vi "rsscope_core_global.vi"() -> ()   [LabVIEW 2018] (continued)
 matches Phase_seg2 specified in the CAN standard.\n\nNote: The maximum sum of Time segment 1 and Time segment 2 is 24.\n\nRemote-control command(s):\nBUS<m>:CAN:T1Segment\nBUS<m>:CAN:T2Segment\n\nAvailable Repeated Capabilities:\nSerialBus: SB1, SB2, SB3, SB4\r\nCANTimeSeg: TS1, TS2\r\n\nRemote-control command(s):\nBUS<m>:CAN:T<CANTimeSeg>Segment"}, {"Level"=4, "Class Only"=FALSE, "Identifier"="RSSCOPE_ATTR_PROTOCOL_CAN_FD_SAMPLE_POINT_ABS", "Descriptive Name"="Protocol CAN FD Sample Point Abs", "Data Type"=0, "Command"="BUS{SerialBus}:CAN:FDAT:T{CANTimeSeg}S", "Access"=2, "Range Table"="RsScope_rngProtocolCANSamplePointAbs", "Read Callback"="", "Write Callback"="", "Supported Models"="", "Instrument Options"="K0|K3", "Flags"=0, "Help"="Set the number of time quanta before the sample point (T1Segment) and after the sample point (T2Segment). T1Segment comprises the segments Synch_seg, Prop_seg, and Phase_seg1 which are specified in the CAN standard. T2Segment matches Phase_seg2 specified in the CAN standard.\n\nNote: The maximum sum of Time segment 1 and Time segment 2 is 24.\n\nRemote-control command(s):\nBUS<m>:CAN:FDATa:T1Segment\nBUS<m>:CAN:FDATa:T2Segment\n\nAvailable Repeated Capabilities:\nSerialBus: SB1, SB2, SB3, SB4\r\nCANTimeSeg: TS1, TS2\r\n\nRemote-control command(s):\nBUS<m>:CAN:FDATa:T<CANTimeSeg>Segment"}, {"Level"=2, "Class Only"=TRUE, "Identifier"="", "Descriptive Name"="FlexRay", "Data Type"=0, "Command"="", "Access"=0, "Range Table"="", "Read Callback"="", "Write Callback"="", "Supported Models"="", "Instrument Options"="", "Flags"=0, "Help"="FlexRay is designed for use in safety-related distributed applications in the automotive industry. It is applied in real-time applications when higher data rates and reliable communication are required. In particular, FlexRay supports x-by-wire applications, e.g. steer-by-wire or brake-by-wire.\n\nAttributes in this class require option R&S RTO-K3."}, {"Level"=3, "Class Only"=FALSE, "Identifier"="RSSCOPE_ATTR_PROTOCOL_FLEXRAY_SOURCE_TYPE", "Descriptive Name"="Protocol FlexRay Source Type", "Data Type"=0, "Command"="BUS{SerialBus}:FLXR:SRCT", "Access"=2, "Range Table"="rsscope_rngFlexRaySrcType", "Read Callback"="", "Write Callback"="", "Supported Models"="", "Instrument Options"="K4", "Flags"=0, "Help"="Selects the FlexRay source type.\n\nAvailable Repeated Capabilities:\nSerialBus: SB1, SB2, SB3, SB4\r\n\nRemote-control command(s):\nBUS<m>:FLXRay:SRCType"}, {"Level"=3, "Class Only"=FALSE, "Identifier"="RSSCOPE_ATTR_PROTOCOL_FLEXRAY_SINGLE_POLARITY", "Descriptive Name"="Protocol FlexRay Single Polarity", "Data Type"=0, "Command"="BUS{SerialBus}:FLXR:POL", "Access"=2, "Range Table"="rsscope_rngFlexRayPolarity", "Read Callback"="", "Write Callback"="", "Supported Models"="", "Instrument Options"="K4", "Flags"=0, "Help"="Selects the wire on which the bus signal is  measured in case of SINGle source type. The setting affects the digitization of the signal.\n\nAvailable Repeated Capabilities:\nSerialBus: SB1, SB2, SB3, SB4\r\n\nRemote-control command(s):\nBUS<m>:FLXRay:POLarity"}, {"Level"=3, "Class Only"=FALSE, "Identifier"="RSSCOPE_ATTR_PROTOCOL_FLEXRAY_SINGLE_PRESET_TRESHOLD", "Descriptive Name"="Protocol FlexRay Single Preset Treshold", "Data Type"=0, "Command"="BUS{SerialBus}:FLXR:PRS", "Access"=2, "Range Table"="rsscope_rngFlexRaySinglePreset", "Read Callback"="", "Write Callback"="", "Supported Models"="", "Instrument Options"="K4", "Flags"=0, "Help"="This control selecs a default threshold voltage.\n\nAvailable Repeated Capabilities:\nSerialBus: SB1, SB2, SB3, SB4\r\n\nRemote-control command(s):\nBUS<m>:FLXRay:PRSingle"}, {"Level"=3, "Class Only"=FALSE, "Identifier"="RSSCOPE_ATTR_PROTOCOL_FLEXRAY_DIFF_PRESET_TRESHOLD", "Descriptive Name"="Protocol FlexRay Differential Preset Treshold", "Data Type"=0, "Command"="BUS{SerialBus}:FLXR:PRD", "Access"=2, "Range Table"="rsscope_rngFlexRayDifferentialPreset", "Read Callback"="", "Write Callback"="", "Supported Models"="", "Instrument Options"="K4", "Flags"=0, "Help"="Selecs a default threshold voltage.\n\nAvailable Repeated Capabilities:\nSerialBus: SB1, SB2, SB3, SB4\r\n\nRemote-control command(s):\nBUS<m>:FLXRay:PRDiff"}, {"Level"=3, "Class Only"=FALSE, "Identifier"="RSSCOPE_ATTR_PROTOCOL_FLEXRAY_THRESHOLD_HIGH", "Descriptive Name"="Protocol FlexRay Threshold High", "Data Type"=1, "Command"="BUS{SerialBus}:FLXR:THR1", "Access"=2, "Range Table"="", "Read Callback"="", "Write Callback"="", "Supported Models"="", "Instrument Options"="K4", "Flags"=0, "Help"="Sets the thresholds for the bus signal if the source type is Single or Differential.\n\nAvailable Repeated Capabilities:\nSerialBus: SB1, SB2, SB3, SB4\r\n\nRemote-control command(s):\nBUS<m>:FLXRay:THReshold<n>"}, {"Level"=3, "Class Only"=FALSE, "Identifier"="RSSCOPE_ATTR_PROTOCOL_FLEXRAY_THRESHOLD_LOW", "Descriptive Name"="Protocol FlexRay Threshold Low", "Data Type"=1, "Command"="BUS{SerialBus}:FLXR:THR2", "Access"=2, "Range Table"="", "Read Callback"="", "Write Callback"="", "Supported Models"="", "Instrument Options"="K4", "Flags"=0, "Help"="Sets the thresholds for the bus signal if the source type is Single or Differential.\n\nAvailable Repeated Capabilities:\nSerialBus: SB1, SB2, SB3, SB4\r\n\nRemote-control command(s):\nBUS<m>:FLXRay:THReshold<n>"}, {"Level"=3, "Class Only"=FALSE, "Identifier"="RSSCOPE_ATTR_PROTOCOL_FLEXRAY_LOGIC_PRESET_TRESHOLD", "Descriptive Name"="Protocol FlexRay Logic Preset Treshold", "Data Type"=0, "Command"="BUS{SerialBus}:FLXR:PRL", "Access"=2, "Range Table"="rsscope_rngFlexRayLogicPreset", "Read Callback"="", "Write Callback"="", "Supported Models"="", "Instrument Options"="K4", "Flags"=0, "Help"="This attribute selecs a default threshold voltage.\n\nAvailable Repeated Capabilities:\nSerialBus: SB1, SB2, SB3, SB4\r\n\nRemote-control command(s):\nBUS<m>:FLXRay:PRLogic"}, {"Level"=3, "Class Only"=FALSE, "Identifier"="RSSCOPE_ATTR_PROTOCOL_FLEXRAY_THRESHOLD_DATA", "Descriptive Name"="Protocol FlexRay Threshold Data", "Data Type"=1, "Command"="BUS{SerialBus}:FLXR:THD", "Access"=2, "Range Table"="rsscope_rngFlexRayLogicTreshold", "Read Callback"="", "Write Callback"="", "Supported Models"="", "Instrument Options"="", "Flags"=0, "Help"="Sets the threshold for the data line if the source type is LOGic.\n\nAvailable Repeated Capabilities:\nSerialBus: SB1, SB2, SB3, SB4\r\n\nRemote-control command(s):\nBUS<m>:FLXRay:THData"}, {"Level"=3, "Class Only"=FALSE, "Identifier"="RSSCOPE_ATTR_PROTOCOL_FLEXRAY_THRESHOLD_ENABLE", "Descriptive Name"="Protocol FlexRay Threshold Enable", "Data Type"=1, "Command"="BUS{SerialBus}:FLXR:THEN", "Access"=2, "Range Table"="rsscope_rngFlexRayLogicTreshold", "Read Callback"="", "Write Callback"="", "Supported Models"="", "Instrument Options"="", "Flags"=0, "Help"="Sets the threshold for the enable line if the source type is LOGic.\n\nAvailable Repeated Capabilities:\nSerialBus: SB1, SB2, SB3, SB4\r\n\nRemote-control command(s):\nBUS<m>:FLXRay:THENable"}, {"Level"=3, "Class Only"=FALSE, "Identifier"="RSSCOPE_ATTR_PROTOCOL_FLEXRAY_BIT_RATE", "Descriptive Name"="Protocol FlexRay Bit Rate", "Data Type"=0, "Command"="BUS{SerialBus}:FLXR:BITR", "Access"=2, "Range Table"="rsscope_rngFlexRayBitRate", "Read Callback"="", "Write Callback"="", "Supported Models"="", "Instrument Options"="", "Flags"=0, "Help"="Selects the bit rate.\n\nAvailable Repeated Capabilities:\nSerialBus: SB1, SB2, SB3, SB4\r\n\nRemote-control command(s):\nBUS<m>:FLXRay:BITRate"}, {"Level"=3, "Class Only"=FALSE, "Identifier"="RSSCOPE_ATTR_PROTOCOL_FLEXRAY_CHANNEL", "Descriptive Name"="Protocol FlexRay Channel", "Data Type"=0, "Command"="BUS{SerialBus}:FLXR:CHTY", "Access"=2, "Range Table"="rsscope_rngFlexRayChannel", "Read Callback"="", "Write Callback"="", "Supported Models"="", "Instrument Options"="K4", "Flags"=0, "Help"="Selects the channel on which the signal is measured. The setting is considered in the calculation of the frame CRC.\n\nAvailable Repeated Capabilities:\nSerialBus: SB1, SB2, SB3, SB4\r\n\nRemote-control command(s):\nBUS<m>:FLXRay:CHTYpe"}, {"Level"=3, "Class Only"=FALSE, "Identifier"="RSSCOPE_ATTR_PROTOCOL_FLEXRAY_SEPARATE_HEADER_BITS", "Descriptive Name"="Protocol FlexRay Separate Header Bits", "Data Type"=3, "Command"="BUS{SerialBus}:FLXR:SEHB", "Access"=2, "Range Table"="", "Read Callback"="", "Write Callback"="", "Supported Models"="", "Instrument Options"="K4", "Flags"=0, "Help"="Affects the decoding and its display. If ON, the leading five indicator bits of the header are decoded as five single bits. Otherwise, the indicator bits are shown as one word with word length five bit.\n\nAvailable Repeated Capabilities:\nSerialBus: SB1, SB2, SB3, SB4\r\n\nRemote-control command(s):\nBUS<m>:FLXRay:SEHB"}, {"Level"=3, "Class Only"=FALSE, "Identifier"="RSSCOPE_ATTR_PROTOCOL_FLEXRAY_SELECTED_FRAME", "Descriptive Name"="Protocol FlexRay Selected Frame", "Data Type"=0, "Command"="", "Access"=2, "Range Table"="", "Read Callback"="", "Write Callback"="", "Supported Models"="", "Instrument Options"="", "Flags"=0, "Help"="Sets selector repeated capability Frame.\n\nAvailable Repeated Capabilities:\nNone\n\nRemote-control command(s):\ncmd"}, {"Level"=3, "Class Only"=FALSE, "Identifier"="RSSCOPE_ATTR_PROTOCOL_FLEXRAY_FRAME_COUNT", "Descriptive Name"="Protocol FlexRay Frame Count", "Data Type"=0, "Command"="BUS{SerialBus}:FLXR:FCO?", "Access"=0, "Range Table"="", "Read Callback"="", "Write Callback"="", "Supported Models"="", "Instrument Options"="K4", "Flags"=0, "Help"="Queries the number of decoded frames.\n\nAvailable Repeated Capabilities:\nSerialBus: SB1, SB2, SB3, SB4\r\n\nRemote-control command(s):\nBUS<m>:FLXRay:FCOunt?"}, {"Level"=3, "Class Only"=FALSE, "Identifier"="RSSCOPE_ATTR_PROTOCOL_FLEXRAY_FRAME_STATUS", "Descriptive Name"="Protocol FlexRay Frame Status", "Data Type"=0, "Command"="BUS{SerialBus}:FLXR:FRAM<Frame>:STAT?", "Access"=0, "Range Table"="rsscope_rngFlexRayFrameStatus", "Read Callback"="rsscope_FormatFlexRayFrameRepCapInt32_ReadCallback.vi", "Write Callback"="", "Supported Models"="", "Instrument Options"="K4", "Flags"=0, "Help"="Returns the overall state of the frame.\n\nAvailable Repeated Capabilities:\nSerialBus: SB1, SB2, SB3, SB4\r\n\nRemote-control command(s):\nBUS<m>:FLXRay:FRAMe<n>:STATus?"}, {"Level"=3, "Class Only"=FALSE, "Identifier"="RSSCOPE_ATTR_PROTOCOL_FLEXRAY_FRAME_START", "Descriptive Name"="Protocol FlexRay Frame Start", "Data Type"=1, "Command"="BUS{SerialBus}:FLXR:FRAM<Frame>:STAR?", "Access"=0, "Range Table"="", "Read Callback"="rsscope_FormatFlexRayFrameRepCapReal64_ReadCallback.vi", "Write Callback"="", "Supported Models"="", "Instrument Options"="K4", "Flags"=0, "Help"="Return the start time of the selected frame.\n\nAvailable Repeated Capabilities:\nSerialBus: SB1, SB2, SB3, SB4\r\n\nRemote-control command(s):\nBUS<m>:FLXRay:FRAMe<n>:STARt?"}, {"Level"=3, "Class Only"=FALSE, "Identifier"="RSSCOPE_ATTR_PROTOCOL_FLEXRAY_FRAME_STOP", "Descriptive Name"="Protocol FlexRay Frame Stop", "Data Type"=1, "Command"="BUS{SerialBus}:FLXR:FRAM<Frame>:STOP?", "Access"=0, "Range Table"="", "Read Callback"="rsscope_FormatFlexRayFrameRepCapReal64_ReadCallback.vi", "Write Callback"="", "Supported Models"="", "Instrument Options"="K4", "Flags"=0, "Help"="Return the stop time of the selected frame.\n\nAvailable Repeated Capabilities:\nSerialBus: SB1, SB2, SB3, SB4\r\n\nRemote-control command(s):\nBUS<m>:FLXRay:FRAMe<n>:STOP?"}, {"Level"=3, "Class Only"=FALSE, "Identifier"="RSSCOPE_ATTR_PROTOCOL_FLEXRAY_FRAME_TYPE", "Descriptive Name"="Protocol FlexRay Frame Type", "Data Type"=0, "Command"="BUS{SerialBus}:FLXR:FRAM<Frame>:TYPE?", "Access"=0, "Range Table"="rsscope_rngFlexRayFrameType", "Read Callback"="rsscope_FormatFlexRayFrameRepCapInt32_ReadCallback.vi", "Write Callback"="", "Supported Models"="", "Instrument Options"="K4", "Flags"=0, "Help"="Returns the frame type of the selected frame.\n\nAvailable Repeated Capabilities:\nSerialBus: SB1, SB2, SB3, SB4\r\n\nRemote-control command(s):\nBUS<m>:FLXRay:FRAMe<n>:TYPE?"}, {"Level"=3, "Class Only"=FALSE, "Identifier"="RSSCOPE_ATTR_PROTOCOL_FLEXRAY_FRAME_FLAGS", "Descriptive Name"="Protocol FlexRay Frame Flags", "Data Type"=0, "Command"="BUS{SerialBus}:FLXR:FRAM<Frame>:FLAG?", "Access"=0, "Range Table"="", "Read Callback"="rsscope_FormatFlexRayFrameRepCapInt32_ReadCallback.vi", "Write Callback"="", "Supported Models"="", "Instrument Options"="K4", "Flags"=0, "Help"="Returns the value of the indicator bits at the beginning of the header segment. The five bits are read as one word.\n\nAvailable Repeated Capabilities:\nSerialBus: SB1, SB2, SB3, SB4\r\n\nRemote-control command(s):\nBUS<m>:FLXRay:FRAMe<n>:FLAGs?"}, {"Level"=3, "Class Only"=FALSE, "Identifier"="RSSCOPE_ATTR_PROTOCOL_FLEXRAY_FRAME_PAYLOAD_LENGTH", "Descriptive Name"="Protocol FlexRay Frame Payload Length", "Data Type"=0, "Command"="BUS{SerialBus}:FLXR:FRAM<Frame>:PAYL?", "Access"=0, "Range Table"="", "Read Callback"="rsscope_FormatFlexRayFrameRepCapInt32_ReadCallback.vi", "Write Callback"="", "Supported Models"="", "Instrument Options"="K4", "Flags"=0, "Help"="Returns the payload length, the number of data words in the payload segment. Information is transmitted in 2-byte words, so the number of data bytes in the payload segment is twice the payload length.\n\nAvailable Repeated Capabilities:\nSerialBus: SB1, SB2, SB3, SB4\r\n\nRemote-control command(s):\nBUS<m>:FLXRay:FRAMe<n>:PAYLength?"}, {"Level"=3, "Class Only"=FALSE, "Identifier"="RSSCOPE_ATTR_PROTOCOL_FLEXRAY_FRAME_IDENTIFIER", "Descriptive Name"="Protocol FlexRay Frame Identifier", "Data Type"=0, "Command"="BUS{SerialBus}:FLXR:FRAM<Frame>:ADID?", "Access"=0, "Range Table"="", "Read Callback"="rsscope_FormatFlexRayFrameRepCapInt32_ReadCallback.vi", "Write Callback"="", "Supported Models"="", "Instrument Options"="K4", "Flags"=0, "Help"="Returns the frame identifier, the number of the slot in which the frame is transmitted.\n\nAvailable Repeated Capabilities:\nSerialBus: SB1, SB2, SB3, SB4\r\n\nRemote-control command(s):\nBUS<m>:FLXRay:FRAMe<n>:ADID?"}, {"Level"=3, "Class Only"=FALSE, "Identifier"="RSSCOPE_ATTR_PROTOCOL_FLEXRAY_FRAME_HEADER_CRC", "Descriptive Name"="Protocol FlexRay Frame Header CRC", "Data Type"=0, "Command"="BUS{SerialBus}:FLXR:FRAM<Frame>:CSV?", "Access"=0, "Range Table"="", "Read Callback"="rsscope_FormatFlexRayFrameRepCapInt32_ReadCallback.vi", "Write Callback"="", "Supported Models"="", "Instrument Options"="K4", "Flags"=0, "Help"="Returns the cyclic redundancy check code of the frame CRC.\n\nAvailable Repeated Capabilities:\nSerialBus: SB1, SB2, SB3, SB4\r\n\nRemote-control command(s):\nBUS<m>:FLXRay:FRAMe<n>:CSValue?"}, {"Level"=3, "Class Only"=FALSE, "Identifier"="RSSCOPE_ATTR_PROTOCOL_FLEXRAY_FRAME_CRC", "Descriptive Name"="Protocol FlexRay Frame CRC", "Data Type"=0, "Command"="BUS{SerialBus}:FLXR:FRAM<Frame>:FCV?", "Access"=0, "Range Table"="", "Read Callback"="rsscope_FormatFlexRayFrameRepCapInt32_ReadCallback.vi", "Write Callback"="", "Supported Models"="", "Instrument Options"="K4", "Flags"=0, "Help"="Returns the checksum value of the header CRC.\n\nAvailable Repeated Capabilities:\nSerialBus: SB1, SB2, SB3, SB4\r\n\nRemote-control command(s):\nBUS<m>:FLXRay:FRAMe<n>:FCValue?"}, {"Level"=3, "Class Only"=FALSE, "Identifier"="RSSCOPE_ATTR_PROTOCOL_FLEXRAY_FRAME_HEADER_CRC_STATUS", "Descriptive Name"="Protocol FlexRay Frame Header CRC Status", "Data Type"=0, "Command"="BUS{SerialBus}:FLXR:FRAM<Frame>:CSST?", "Access"=0, "Range Table"="rsscope_rngFlexRayFieldStatus", "Read Callback"="rsscope_FormatFlexRayFrameRepCapInt32_ReadCallback.vi", "Write Callback"="", "Supported Models"="", "Instrument Options"="K4", "Flags"=0, "Help"="Returns the state of the cyclic redundancy check code of the frame data.\n\nAvailable Repeated Capabilities:\nSerialBus: SB1, SB2, SB3, SB4\r\n\nRemote-control command(s):\nBUS<m>:FLXRay:FRAMe<n>:CSSTate?"}, {"Level"=3, "Class Only"=FALSE, "Identifier"="RSSCOPE_ATTR_PROTOCOL_FLEXRAY_FRAME_CRC_STATUS", "Descriptive Name"="Protocol FlexRay Frame CRC Status", "Data Type"=0, "Command"="BUS{SerialBus}:FLXR:FRAM<Frame>:FCST?", "Access"=0, "Range Table"="rsscope_rngFlexRayFieldStatus", "Read Callback"="rsscope_FormatFlexRayFrameRepCapInt32_ReadCallback.vi", "Write Callback"="", "Supported Models"="", "Instrument Options"="K4", "Flags"=0, "Help"="Returns the state of the cyclic redundancy check code of the header data.\n\nAvailable Repeated Capabilities:\nSerialBus: SB1, SB2, SB3, SB4\r\n\nRemote-control command(s):\nBUS<m>:FLXRay:FRAMe<n>:FCSTate?"}, {"Level"=3, "Class Only"=FALSE, "Identifier"="RSSCOPE_ATTR_PROTOCOL_FLEXRAY_FRAME_LABEL", "Descriptive Name"="Protocol FlexRay Frame Label", "Data Type"=2, "Command"="BUS{SerialBus}:FLXR:FRAM<Frame>:SYMB?", "Access"=0, "Range Table"="", "Read Callback"="rsscope_FormatFlexRayFrameRepCapString_ReadCallback.vi", "Write Callback"="", "Supported Models"="", "Instrument Options"="K4", "Flags"=0, "Help"="This attribute returns the symbolic label of the specified frame if the label list is enabled.\n\nAvailable Repeated Capabilities:\nSerialBus: SB1, SB2, SB3, SB4\r\n\nRemote-control command(s):\nBUS<m>:FLXRay:FRAMe<n>:SYMBol?"}, {"Level"=3, "Class Only"=TRUE, "Identifier"="", "Descriptive Name"="Line", "Data Type"=0, "Command"="", "Access"=0, "Range Table"="", "Read Callback"="", "Write Callback"="", "Supported Models"="", "Instrument Options"="", "Flags"=0, "Help"="Selects Flex Ray Line."}, {"Level"=4, "Class Only"=FALSE, "Identifier"="RSSCOPE_ATTR_PROTOCOL_FLEXRAY_SOURCE", "Descriptive Name"="Protocol FlexRay Source", "Data Type"=0, "Command"="BUS{SerialBus}:FLXR:SOUR{Line}", "Access"=2, "Range Table"="rsscope_rngProtocolWaveformSource", "Read Callback"="", "Write Callback"="", "Supported Models"="", "Instrument Options"="K4", "Flags"=0, "Help"="Selects the source of the waveform.\n\nAvailable Repeated Capabilities:\nSerialBus: SB1, SB2, SB3, SB4\r\nLine: Data, Enable\r\n\nRemote-control command(s):\nBUS<m>:FLXRay:SOURce<n>"}, {"Level"=2, "Class Only"=TRUE, "Identifier"="", "Descriptive Name"="Audio Signals", "Data Type"=0, "Command"="", "Access"=0, "Range Table"="", "Read Callback"="", "Write Callback"="", "Supported Models"="", "Instrument Options"="", "Flags"=0, "Help"="This class contains attributes that configure and analyze audio signals."}, {"Level"=3, "Class Only"=FALSE, "Identifier"="RSSCOPE_ATTR_PROTOCOL_AUDIO_VARIANT", "Descriptive Name"="Protocol Audio Variant", "Data Type"=0, "Command"="BUS{SerialBus}:I2S:AVAR", "Access"=2, "Range Table"="rsscope_rngAudioVariant", "Read Callback"="", "Write Callback"="", "Supported Models"="", "Instrument Options"="", "Flags"=0, "Help"="Selects the audio signal type.\n\nAvailable Repeated Capabilities:\nSerialBus: SB1, SB2, SB3, SB4\r\n\nRemote-control command(s):\nBUS<m>:I2S:AVARiant"}, {"Level"=3, "Class Only"=FALSE, "Identifier"="RSSCOPE_ATTR_PROTOCOL_AUDIO_TRESHOLDS_COUPLING", "Descriptive Name"="Protocol Audio Tresholds Coupling", "Data Type"=3, "Command"="BUS{SerialBus}:I2S:TCO", "Access"=2, "Range Table"="", "Read Callback"="", "Write Callback"="", "Supported Models"="", "Instrument Options"="", "Flags"=0, "Help"="Enables or disables tresholds coupling.\n\nAvailable Repeated Capabilities:\nSerialBus: SB1, SB2, SB3, SB4\r\n\nRemote-control command(s):\nBUS<m>:I2S:TCOupling"}, {"Level"=3, "Class Only"=FALSE, "Identifier"="RSSCOPE_ATTR_PROTOCOL_AUDIO_WORD_LENGTH", "Descriptive Name"="Protocol Audio Word Length", "Data Type"=0, "Command"="BUS{SerialBus}:I2S:WLEN", "Access"=2, "Range Table"="rsscope_rngAudioLength", "Read Callback"="", "Write Callback"="", "Supported Models"="", "Instrument Options"="", "Flags"=0, "Help"="Defines the number of bits in an audio data word.\n\nAvailable Repeated Capabilities:\nSerialBus: SB1, SB2, SB3, SB4\r\n\nRemote-control command(s):\nBUS<m>:I2S:WLENgth"}, {"Level"=3, "Class Only"=FALSE, "Identifier"="RSSCOPE_ATTR_PROTOCOL_AUDIO_CHANNEL_ORDER", "Descriptive Name"="Protocol Audio Channel Order", "Data Type"=0, "Command"="BUS{SerialBus}:I2S:CHAN:ORD", "Access"=2, "Range Table"="rsscope_rngAudioChannelOrder", "Read Callback"="", "Write Callback"="", "Supported Models"="", "Instrument Options"="", "Flags"=0, "Help"="Defines if the left or the right channel is the first channel in the frame.\n\nAvailable Repeated Capabilities:\nSerialBus: SB1, SB2, SB3, SB4\r\n\nRemote-control command(s):\nBUS<m>:I2S:CHANnel:ORDer"}, {"Level"=3, "Class Only"=FALSE, "Identifier"="RSSCOPE_ATTR_PROTOCOL_AUDIO_BIT_ORDER", "Descriptive Name"="Protocol Audio Bit Order", "Data Type"=0, "Command"="BUS{SerialBus}:I2S:BORD", "Access"=2, "Range Table"="rsscope_rngProtocolAudioBitOrder", "Read Callback"="", "Write Callback"="", "Supported Models"="", "Instrument Options"="", "Flags"=0, "Help"="Select if the data of the messages starts with msb or lsb.\n\nAvailable Repeated Capabilities:\nSerialBus: SB1, SB2, SB3, SB4\r\n\nRemote-control command(s):\nBUS<m>:I2S:BORDer"}, {"Level"=3, "Class Only"=FALSE, "Identifier"="RSSCOPE_ATTR_PROTOCOL_AUDIO_CHANNEL_OFFSET", "Descriptive Name"="Protocol Audio Channel Offset", "Data Type"=0, "Command"="BUS{SerialBus}:I2S:CHAN:OFFS", "Access"=2, "Range Table"="rsscope_rngAudioOffset", "Read Callback"="", "Write Callback"="", "Supported Models"="", "Instrument Options"="", "Flags"=0, "Help"="Sets the number of bits between the channel start and the start of the audio word. The setting is available for left-justified data format and TDM audio signals.\n\nAvailable Repeated Capabilities:\nSerialBus: SB1, SB2, SB3, SB4\r\n\nRemote-control command(s):\nBUS<m>:I2S:CHANnel:OFFSet"}, {"Level"=3, "Class Only"=FALSE, "Identifier"="RSSCOPE_ATTR_PROTOCOL_AUDIO_CHANNEL_LENGTH", "Descriptive Name"="Protocol Audio Channel Length", "Data Type"=0, "Command"="BUS{SerialBus}:I2S:CHAN:LENG", "Access"=2, "Range Table"="rsscope_rngAudioLength", "Read Callback"="", "Write Callback"="", "Supported Models"="", "Instrument Options"="", "Flags"=0, "Help"="Sets the number of bits in a channel block for right-justified data format and TDM audio signals.\n\nAvailable Repeated Capabilities:\nSerialBus: SB1, SB2, SB3, SB4\r\n\nRemote-control command(s):\nBUS<m>:I2S:CHANnel:LENGth"}, {"Level"=3, "Class Only"=FALSE, "Identifier"="RSSCOPE_ATTR_PROTOCOL_AUDIO_FRAME_OFFSET", "Descriptive Name"="Protocol Audio Frame Offset", "Data Type"=0, "Command"="BUS{SerialBus}:I2S:FOFF", "Access"=2, "Range Table"="rsscope_rnglAudioFrameOffset", "Read Callback"="", "Write Callback"="", "Supported Models"="", "Instrument Options"="", "Flags"=0, "Help"="Sets the number of bits between the frame start and the start of the first channel of a TDM audio line. Each FSYNC edge restarts the offset count.\n\nAvailable Repeated Capabilities:\nSerialBus: SB1, SB2, SB3, SB4\r\n\nRemote-control command(s):\nBUS<m>:I2S:FOFFset"}, {"Level"=3, "Class Only"=FALSE, "Identifier"="RSSCOPE_ATTR_PROTOCOL_AUDIO_TDM_CHANNELS", "Descriptive Name"="Protocol Audio TDM Channels", "Data Type"=0, "Command"="BUS{SerialBus}:I2S:CHAN:TDMC", "Access"=2, "Range Table"="rsscope_rngAudioTDMChannels", "Read Callback"="", "Write Callback"="", "Supported Models"="", "Instrument Options"="", "Flags"=0, "Help"="Sets the number of channels transmitted on the TDM audio line.\n\nAvailable Repeated Capabilities:\nSerialBus: SB1, SB2, SB3, SB4\r\n\nRemote-control command(s):\nBUS<m>:I2S:CHANnel:TDMCount"}, {"Level"=3, "Class Only"=FALSE, "Identifier"="RSSCOPE_ATTR_PROTOCOL_AUDIO_SELECTED_FRAME", "Descriptive Name"="Protocol Audio Selected Frame", "Data Type"=0, "Command"="", "Access"=2, "Range Table"="", "Read Callback"="", "Write Callback"="", "Supported Models"="", "Instrument Options"="", "Flags"=0, "Help"="Sets selector repeated capability Frame.\n\nAvailable Repeated Capabilities:\nNone\n\nRemote-control command(s):\ncmd"}, {"Level"=3, "Class Only"=FALSE, "Identifier"="RSSCOPE_ATTR_PROTOCOL_AUDIO_FRAME_COUNT", "Descriptive Name"="Protocol Audio Frame Count", "Data Type"=0, "Command"="BUS{SerialBus}:I2S:FCO?", "Access"=0, "Range Table"="", "Read Callback"="", "Write Callback"="", "Supported Models"="", "Instrument Options"="", "Flags"=0, "Help"="Queries the number of decoded frames.\n\nAvailable Repeated Capabilities:\nSerialBus: SB1, SB2, SB3, SB4\r\n\nRemote-control command(s):\nBUS<m>:I2S:FCOunt?"}, {"Level"=3, "Class Only"=TRUE, "Identifier"="", "Descriptive Name"="TDM Channel", "Data Type"=0, "Command"="", "Access"=0, "Range Table"="", "Read Callback"="", "Write Callback"="", "Supported Models"="", "Instrument Options"="", "Flags"=0, "Help"="This class contains attributes with TDMChannel repeated capability."}, {"Level"=3, "Class Only"=TRUE, "Identifier"="", "Descriptive Name"="Clock", "Data Type"=0, "Command"="", "Access"=0, "Range Table"="", "Read Callback"="", "Write Callback"="", "Supported Models"="", "Instrument Options"="", "Flags"=0, "Help"="Configures the clock line properties."}, {"Level"=4, "Class Only"=FALSE, "Identifier"="RSSCOPE_ATTR_PROTOCOL_AUDIO_CLOCK_SOURCE", "Descriptive Name"="Protocol Audio Clock Source", "Data Type"=0, "Command"="BUS{SerialBus}:I2S:CLOC:SOUR", "Access"=2, "Range Table"="rsscope_rngProtocolWaveformSource", "Read Callback"="", "Write Callback"="", "Supported Models"="", "Instrument Options"="", "Flags"=0, "Help"="Selects the source of the waveform.\n\nAvailable Repeated Capabilities:\nSerialBus: SB1, SB2, SB3, SB4\r\n\nRemote-control command(s):\nBUS<m>:I2S:CLOCk:SOURce"}, {"Level"=4, "Class Only"=FALSE, "Identifier"="RSSCOPE_ATTR_PROTOCOL_AUDIO_CLOCK_THRESHOLD", "Descriptive Name"="Protocol Audio Clock Threshold", "Data Type"=1, "Command"="BUS{SerialBus}:I2S:CLOC:THR", "Access"=2, "Range Table"="rsscope_rngAudioTreshold", "Read Callback"="", "Write Callback"="", "Supported Models"="", "Instrument Options"="", "Flags"=0, "Help"="Sets the threshold value for the clock line SCLK.\n\nAvailable Repeated Capabilities:\nSerialBus: SB1, SB2, SB3, SB4\r\n\nRemote-control command(s):\nBUS<m>:I2S:CLOCk:THReshold"}, {"Level"=4, "Class Only"=FALSE, "Identifier"="RSSCOPE_ATTR_PROTOCOL_AUDIO_CLOCK_POLARITY", "Descriptive Name"="Protocol Audio Clock Polarity", "Data Type"=0, "Command"="BUS{SerialBus}:I2S:CLOC:POL", "Access"=2, "Range Table"="rsscope_rngAudioClockPolarity", "Read Callback"="", "Write Callback"="", "Supported Models"="", "Instrument Options"="", "Flags"=0, "Help"="Selects line polarity.\n\nAvailable Repeated Capabilities:\nSerialBus: SB1, SB2, SB3, SB4\r\n\nRemote-control command(s):\nBUS<m>:I2S:CLOCk:POLarity"}, {"Level"=3, "Class Only"=TRUE, "Identifier"="", "Descriptive Name"="Word Select", "Data Type"=0, "Command"="", "Access"=0, "Range Table"="", "Read Callback"="", "Write Callback"="", "Supported Models"="", "Instrument Options"="", "Flags"=0, "Help"="Configures the word select line properties for I2S standard"}, {"Level"=4, "Class Only"=FALSE, "Identifier"="RSSCOPE_ATTR_PROTOCOL_AUDIO_WS_SOURCE", "Descriptive Name"="Protocol Audio WS Source", "Data Type"=0, "Command"="BUS{SerialBus}:I2S:WSEL:SOUR", "Access"=2, "Range Table"="rsscope_rngProtocolWaveformSource", "Read Callback"="", "Write Callback"="", "Supported Models"="", "Instrument Options"="", "Flags"=0, "Help"="Selects the source of the word select line for I2S standard, left- und right-justified data formats, or the source of the frame synchronization pulse for TDM audio signals.\n\nAvailable Repeated Capabilities:\nSerialBus: SB1, SB2, SB3, SB4\r\n\nRemote-control command(s):\nBUS<m>:I2S:WSELect:SOURce"}, {"Level"=4, "Class Only"=FALSE, "Identifier"="RSSCOPE_ATTR_PROTOCOL_AUDIO_WS_THRESHOLD", "Descriptive Name"="Protocol Audio WS Threshold", "Data Type"=1, "Command"="BUS{SerialBus}:I2S:WSEL:THR", "Access"=2, "Range Table"="rsscope_rngAudioTreshold", "Read Callback"="", "Write Callback"="", "Supported Models"="", "Instrument Options"="", "Flags"=0, "Help"="Sets the threshold value for the word select and FSYNC lines.\n\nAvailable Repeated Capabilities:\nSerialBus: SB1, SB2, SB3, SB4\r\n\nRemote-control command(s):\nBUS<m>:I2S:WSELect:THReshold"}, {"Level"=4, "Class Only"=FALSE, "Identifier"="RSSCOPE_ATTR_PROTOCOL_AUDIO_WS_POLARITY", "Descriptive Name"="Protocol Audio WS Polarity", "Data Type"=0, "Command"="BUS{SerialBus}:I2S:WSEL:POL", "Access"=2, "Range Table"="rsscope_rngAudioWSPolarity", "Read Callback"="", "Write Callback"="", "Supported Models"="", "Instrument Options"="", "Flags"=0, "Help"="Selects line polarity.\n\nAvailable Repeated Capabilities:\nSerialBus: SB1, SB2, SB3, SB4\r\n\nRemote-control command(s):\nBUS<m>:I2S:WSELect:POLarity"}, {"Level"=3, "Class Only"=TRUE, "Identifier"="", "Descriptive Name"="Data", "Data Type"=0, "Command"="", "Access"=0, "Range Table"="", "Read Callback"="", "Write Callback"="", "Supported Models"="", "Instrument Options"="", "Flags"=0, "Help"="Configures properties of the audio data line."}, {"Level"=4, "Class Only"=FALSE, "Identifier"="RSSCOPE_ATTR_PROTOCOL_AUDIO_DATA_SOURCE", "Descriptive Name"="Protocol Audio Data Source", "Data Type"=0, "Command"="BUS{SerialBus}:I2S:DATA:SOUR", "Access"=2, "Range Table"="rsscope_rngProtocolWaveformSource", "Read Callback"="", "Write Callback"="", "Supported Models"="", "Instrument Options"="", "Flags"=0, "Help"="Selects the source of the audio data line.\n\nAvailable Repeated Capabilities:\nSerialBus: SB1, SB2, SB3, SB4\r\n\nRemote-control command(s):\nBUS<m>:I2S:DATA:SOURce"}, {"Level"=4, "Class Only"=FALSE, "Identifier"="RSSCOPE_ATTR_PROTOCOL_AUDIO_DATA_THRESHOLD", "Descriptive Name"="Protocol Audio Data Threshold", "Data Type"=1, "Command"="BUS{SerialBus}:I2S:DATA:THR", "Access"=2, "Range Table"="rsscope_rngAudioTreshold", "Read Callback"="", "Write Callback"="", "Supported Models"="", "Instrument Options"="", "Flags"=0, "Help"="Sets the threshold value for the data line.\n\nAvailable Repeated Capabilities:\nSerialBus: SB1, SB2, SB3, SB4\r\n\nRemote-control command(s):\nBUS<m>:I2S:DATA:THReshold"}, {"Level"=4, "Class Only"=FALSE, "Identifier"="RSSCOPE_ATTR_PROTOCOL_AUDIO_DATA_POLARITY", "Descriptive Name"="Protocol Audio Data Polarity", "Data Type"=0, "Command"="BUS{SerialBus}:I2S:DATA:POL", "Access"=2, "Range Table"="rsscope_rngProtocolSPIPolarity", "Read Callback"="", "Write Callback"="", "Supported Models"="", "Instrument Options"="", "Flags"=0, "Help"="Selects line polarity.\n\nAvailable Repeated Capabilities:\nSerialBus: SB1, SB2, SB3, SB4\r\n\nRemote-control command(s):\nBUS<m>:I2S:DATA:POLarity"}, {"Level"=3, "Class Only"=TRUE, "Identifier"="", "Descriptive Name"="Track", "Data Type"=0, "Command"="", "Access"=0, "Range Table"="", "Read Callback"="", "Write Callback"="", "Supported Models"="", "Instrument Options"="", "Flags"=0, "Help"="This class contains methods for enabling and disabling waveform tracks."}, {"Level"=4, "Class Only"=FALSE, "Identifier"="RSSCOPE_ATTR_PROTOCOL_AUDIO_TRACK_LEFT_ENABLED", "Descriptive Name"="Protocol Audio Track Left Enabled", "Data Type"=3, "Command"="BUS{SerialBus}:I2S:TRAC:LEFT", "Access"=2, "Range Table"="", "Read Callback"="", "Write Callback"="", "Supported Models"="", "Instrument Options"="", "Flags"=0, "Help"="Enables or disables the track of the indicated channel. The attribute is relevant for I2S standard, left-justified audio data formats.\n\nAvailable Repeated Capabilities:\nSerialBus: SB1, SB2, SB3, SB4\r\n\nRemote-control command(s):\nBUS<m>:I2S:TRACk:LEFT"}, {"Level"=4, "Class Only"=FALSE, "Identifier"="RSSCOPE_ATTR_PROTOCOL_AUDIO_TRACK_RIGHT_ENABLED", "Descriptive Name"="Protocol Audio Track Right Enabled", "Data Type"=3, "Command"="BUS{SerialBus}:I2S:TRAC:RIGH", "Access"=2, "Range Table"="", "Read Callback"="", "Write Callback"="", "Supported Models"="", "Instrument Options"="", "Flags"=0, "Help"="Enables or disables the track of the indicated channel. The attribute is  relevant for I2S standard, right-justified audio data formats.\n\nAvailable Repeated Capabilities:\nSerialBus: SB1, SB2, SB3, SB4\r\n\nRemote-control command(s):\nBUS<m>:I2S:TRACk:RIGHt"}, {"Level"=4, "Class Only"=FALSE, "Identifier"="RSSCOPE_ATTR_PROTOCOL_AUDIO_TRACK_TDM_CHANNEL_ENABLED", "Descriptive Name"="Protocol Audio Track TDM Channel Enabled", "Data Type"=3, "Command"="BUS{SerialBus}:I2S:TRAC:TD{TDMChannel}C", "Access"=2, "Range Table"="", "Read Callback"="", "Write Callback"="", "Supported Models"="", "Instrument Options"="", "Flags"=0, "Help"="Enables or disables the track of the indicated channel. The attribute is relevant for TDM audio data.\n\nAvailable Repeated Capabilities:\nSerialBus: SB1, SB2, SB3, SB4\r\nTDMChannel: TDM1, TDM2, TDM3, TDM4, TDM5, TDM6, TDM7, TDM8\r\n\nRemote-control command(s):\nBUS<m>:I2S:TRACk:TD<TDMChannel>Ch"}, {"Level"=2, "Class Only"=TRUE, "Identifier"="", "Descriptive Name"="MIL1553", "Data Type"=0, "Command"="", "Access"=0, "Range Table"="", "Read Callback"="", "Write Callback"="", "Supported Models"="", "Instrument Options"="", "Flags"=0, "Help"="MIL-1553 (Option R&S RTO-K6)"}, {"Level"=3, "Class Only"=FALSE, "Identifier"="RSSCOPE_ATTR_PROTOCOL_MIL1553_SOURCE", "Descriptive Name"="Protocol MIL1553 Source", "Data Type"=0, "Command"="BUS{SerialBus}:MILS:SOUR", "Access"=2, "Range Table"="rsscope_rngProtocolDataSource", "Read Callback"="", "Write Callback"="", "Supported Models"="RTO|RTP", "Instrument Options"="", "Flags"=0, "Help"="Sets the channel for the signal source.\n\nAvailable Repeated Capabilities:\nSerialBus: SB1, SB2, SB3, SB4\r\n\nRemote-control command(s):\nBUS<m>:MILStd:SOURce"}, {"Level"=3, "Class Only"=FALSE, "Identifier"="RSSCOPE_ATTR_PROTOCOL_MIL1553_POLARITY", "Descriptive Name"="Protocol MIL1553 Polarity", "Data Type"=0, "Command"="BUS{SerialBus}:MILS:POL", "Access"=2, "Range Table"="rsscope_rngProtocolMIL1553Polarity", "Read Callback"="", "Write Callback"="", "Supported Models"="RTO|RTP", "Instrument Options"="", "Flags"=0, "Help"="Selects the wire on which the bus signal is measured.\n\nAvailable Repeated Capabilities:\nSerialBus: SB1, SB2, SB3, SB4\r\n\nRemote-control command(s):\nBUS<m>:MILStd:POLarity"}, {"Level"=3, "Class Only"=FALSE, "Identifier"="RSSCOPE_ATTR_PROTOCOL_MIL1553_THRESHOLD_HIGH", "Descriptive Name"="Protocol MIL1553 Threshold High", "Data Type"=1, "Command"="BUS{SerialBus}:MILS:THR:HIGH", "Access"=2, "Range Table"="rsscope_rngProtocolMIL1553ThresholdHigh", "Read Callback"="", "Write Callback"="", "Supported Models"="RTO|RTP", "Instrument Options"="", "Flags"=0, "Help"="Sets the lower threshold level of the signal.\n\nAvailable Repeated Capabilities:\nSerialBus: SB1, SB2, SB3, SB4\r\n\nRemote-control command(s):\nBUS<m>:MILStd:THReshold:HIGH"}, {"Level"=3, "Class Only"=FALSE, "Identifier"="RSSCOPE_ATTR_PROTOCOL_MIL1553_THRESHOLD_LOW", "Descriptive Name"="Protocol MIL1553 Threshold Low", "Data Type"=1, "Command"="BUS{SerialBus}:MILS:THR:LOW", "Access"=2, "Range Table"="rsscope_rngProtocolMIL1553ThresholdLow", "Read Callback"="", "Write Callback"="", "Supported Models"="RTO|RTP", "Instrument Options"="", "Flags"=0, "Help"="Sets the lower threshold level of the signal.\n\nAvailable Repeated Capabilities:\nSerialBus: SB1, SB2, SB3, SB4\r\n\nRemote-control command(s):\nBUS<m>:MILStd:THReshold:LOW"}, {"Level"=3, "Class Only"=FALSE, "Identifier"="RSSCOPE_ATTR_PROTOCOL_MIL1553_THRESHOLD_PRESET", "Descriptive Name"="Protocol MIL1553 Threshold Preset", "Data Type"=0, "Command"="BUS{SerialBus}:MILS:PRES", "Access"=2, "Range Table"="rsscope_rngProtocolMIL1553ThresholdPreset", "Read Callback"="", "Write Callback"="", "Supported Models"="RTO|RTP", "Instrument Options"="", "Flags"=0, "Help"="Sets the default threshold voltage.\n\nAvailable Repeated Capabilities:\nSerialBus: SB1, SB2, SB3, SB4\r\n\nRemote-control command(s):\nBUS<m>:MILStd:PRESet"}, {"Level"=3, "Class Only"=TRUE, "Identifier"="", "Descriptive Name"="Timing", "Data Type"=0, "Command"="", "Access"=0, "Range Table"="", "Read Callback"="", "Write Callback"="", "Supported Models"="", "Instrument Options"="", "Flags"=0, "Help"="Specifies the ranges of the timeouts."}, {"Level"=4, "Class Only"=FALSE, "Identifier"="RSSCOPE_ATTR_PROTOCOL_MIL1553_MIN_GAP_ENABLED", "Descriptive Name"="Protocol MIL1553 Min Gap Enabled", "Data Type"=3, "Command"="BUS{SerialBus}:MILS:MING:SEL", "Access"=2, "Range Table"="", "Read Callback"="", "Write Callback"="", "Supported Models"="RTO|RTP", "Instrument Options"="", "Flags"=0, "Help"="Enables the selection of the min gap.\n\nAvailable Repeated Capabilities:\nSerialBus: SB1, SB2, SB3, SB4\r\n\nRemote-control command(s):\nBUS<m>:MILStd:MINGap:SELect"}, {"Level"=4, "Class Only"=FALSE, "Identifier"="RSSCOPE_ATTR_PROTOCOL_MIL1553_MIN_GAP_TIME", "Descriptive Name"="Protocol MIL1553 Min Gap Time", "Data Type"=1, "Command"="BUS{SerialBus}:MILS:MING:BITS", "Access"=2, "Range Table"="rsscope_rngProtocolMIL1553MinGapTime", "Read Callback"="", "Write Callback"="", "Supported Models"="RTO|RTP", "Instrument Options"="", "Flags"=0, "Help"="Sets a value for the min timing gap between two words.\n\nAvailable Repeated Capabilities:\nSerialBus: SB1, SB2, SB3, SB4\r\n\nRemote-control command(s):\nBUS<m>:MILStd:MINGap:BITS"}, {"Level"=4, "Class Only"=FALSE, "Identifier"="RSSCOPE_ATTR_PROTOCOL_MIL1553_MAX_RESPONSE_ENABLED", "Descriptive Name"="Protocol MIL1553 Max Response Enabled", "Data Type"=3, "Command"="BUS{SerialBus}:MILS:MAXR:SEL", "Access"=2, "Range Table"="", "Read Callback"="", "Write Callback"="", "Supported Models"="RTO|RTP", "Instrument Options"="", "Flags"=0, "Help"="Enables the selection of the max gap.\n\nAvailable Repeated Capabilities:\nSerialBus: SB1, SB2, SB3, SB4\r\n\nRemote-control command(s):\nBUS<m>:MILStd:MAXResponse:SELect"}, {"Level"=4, "Class Only"=FALSE, "Identifier"="RSSCOPE_ATTR_PROTOCOL_MIL1553_MAX_RESPONSE_TIME", "Descriptive Name"="Protocol MIL1553 Max Response Time", "Data Type"=1, "Command"="BUS{SerialBus}:MILS:MAXR:BITS", "Access"=2, "Range Table"="rsscope_rngProtocolMIL1553MaxResponseTime", "Read Callback"="", "Write Callback"="", "Supported Models"="RTO|RTP", "Instrument Options"="", "Flags"=0, "Help"="Sets the value for the maximum response time.\n\nAvailable Repeated Capabilities:\nSerialBus: SB1, SB2, SB3, SB4\r\n\nRemote-control command(s):\nBUS<m>:MILStd:MAXResponse:BITS"}, {"Level"=3, "Class Only"=TRUE, "Identifier"="", "Descriptive Name"="Decoding Results", "Data Type"=0, "Command"="", "Access"=0, "Range Table"="", "Read Callback"="", "Write Callback"="", "Supported Models"="", "Instrument Options"="", "Flags"=0, "Help"="Returns the decoding result of the specified word."}, {"Level"=4, "Class Only"=FALSE, "Identifier"="RSSCOPE_ATTR_PROTOCOL_MIL1553_DECODING_RESULTS_WORDS_COUNT", "Descriptive Name"="Protocol MIL1553 Decoding Results Words Count", "Data Type"=0, "Command"="BUS{SerialBus}:MILS:WCO?", "Access"=0, "Range Table"="", "Read Callback"="", "Write Callback"="", "Supported Models"="RTO|RTP", "Instrument Options"="", "Flags"=0, "Help"="Returns the number of decoded words.\n\nAvailable Repeated Capabilities:\nSerialBus: SB1, SB2, SB3, SB4\r\n\nRemote-control command(s):\nBUS<m>:MILStd:WCOunt?"}, {"Level"=2, "Class Only"=TRUE, "Identifier"="", "Descriptive Name"="ARINC429", "Data Type"=0, "Command"="", "Access"=0, "Range Table"="", "Read Callback"="", "Write Callback"="", "Supported Models"="", "Instrument Options"="", "Flags"=0, "Help"="ARINC 429 (Option R&S RTO-K7)"}, {"Level"=3, "Class Only"=FALSE, "Identifier"="RSSCOPE_ATTR_PROTOCOL_ARINC429_SOURCE", "Descriptive Name"="Protocol ARINC429 Source", "Data Type"=0, "Command"="BUS{SerialBus}:ARIN:SOUR", "Access"=2, "Range Table"="rsscope_rngProtocolDataSource", "Read Callback"="", "Write Callback"="", "Supported Models"="RTO|RTP", "Instrument Options"="", "Flags"=0, "Help"="Sets the channel for the signal source.\n\nAvailable Repeated Capabilities:\nSerialBus: SB1, SB2, SB3, SB4\r\n\nRemote-control command(s):\nBUS<m>:ARINc:SOURce"}, {"Level"=3, "Class Only"=FALSE, "Identifier"="RSSCOPE_ATTR_PROTOCOL_ARINC429_POLARITY", "Descriptive Name"="Protocol ARINC429 Polarity", "Data Type"=0, "Command"="BUS{SerialBus}:ARIN:POL", "Access"=2, "Range Table"="rsscope_rngProtocolARINC429Polarity", 
